vi "Actor Core.vi"(8 "error in":errorcluster, 11 "UI Main in":refnum<class "UI Main.lvclass">) -> (0 "error out":errorcluster, 3 "Actor out":refnum<class "Actor.lvclass">)   [LabVIEW 2020, in "UI Main.lvlib" / "UI Main.lvclass"]
doc: "(<B>Filename</B>: Actor Framework.lvlib:Actor.lvclass:Actor Core.vi)\n\nReceives messages to the actor, reacts to them, and initiates any error handling that may shut the actor down.\n\nDescendant classes may override this VI to append parallel tasks for the actor to complete while it handles messages. Overrides use the Call Parent Class Method node."
uses:
  UI Main.lvclass
  C:/Program Files (x86)/National Instruments/LabVIEW 2020/vi.lib/ActorFramework/Actor/Actor.lvclass
  <vilib>/ActorFramework/Actor/Actor.lvclass
  UI Status/UI Status/UI Status.lvclass
  UI Main Startup/UI Main Startup/UI Main Startup.lvclass
  <vilib>/ActorFramework/Actor/Actor.lvclass/Actor.ctl
  <vilib>/ActorFramework/Message Enqueuer/Message Enqueuer.lvclass/Message Enqueuer.ctl
  UI Main.lvclass/UI Main.ctl
  <vilib>/ActorFramework/Message Enqueuer/Init from Existing Queue.vi
  <vilib>/ActorFramework/Message Enqueuer/Enqueue.vi
  <vilib>/ActorFramework/Stop Msg/Stop Msg.lvclass
  C:/Program Files (x86)/National Instruments/LabVIEW 2020/vi.lib/ActorFramework/Message/Message.lvclass
  <vilib>/ActorFramework/Message Priority Queue/Priority Enqueue.vi
  <vilib>/ActorFramework/Message Enqueuer/Message Enqueuer.lvclass
  C:/git/Personal/Sandbox/ActorProject/UI Main/UI Main/UI Main.lvclass
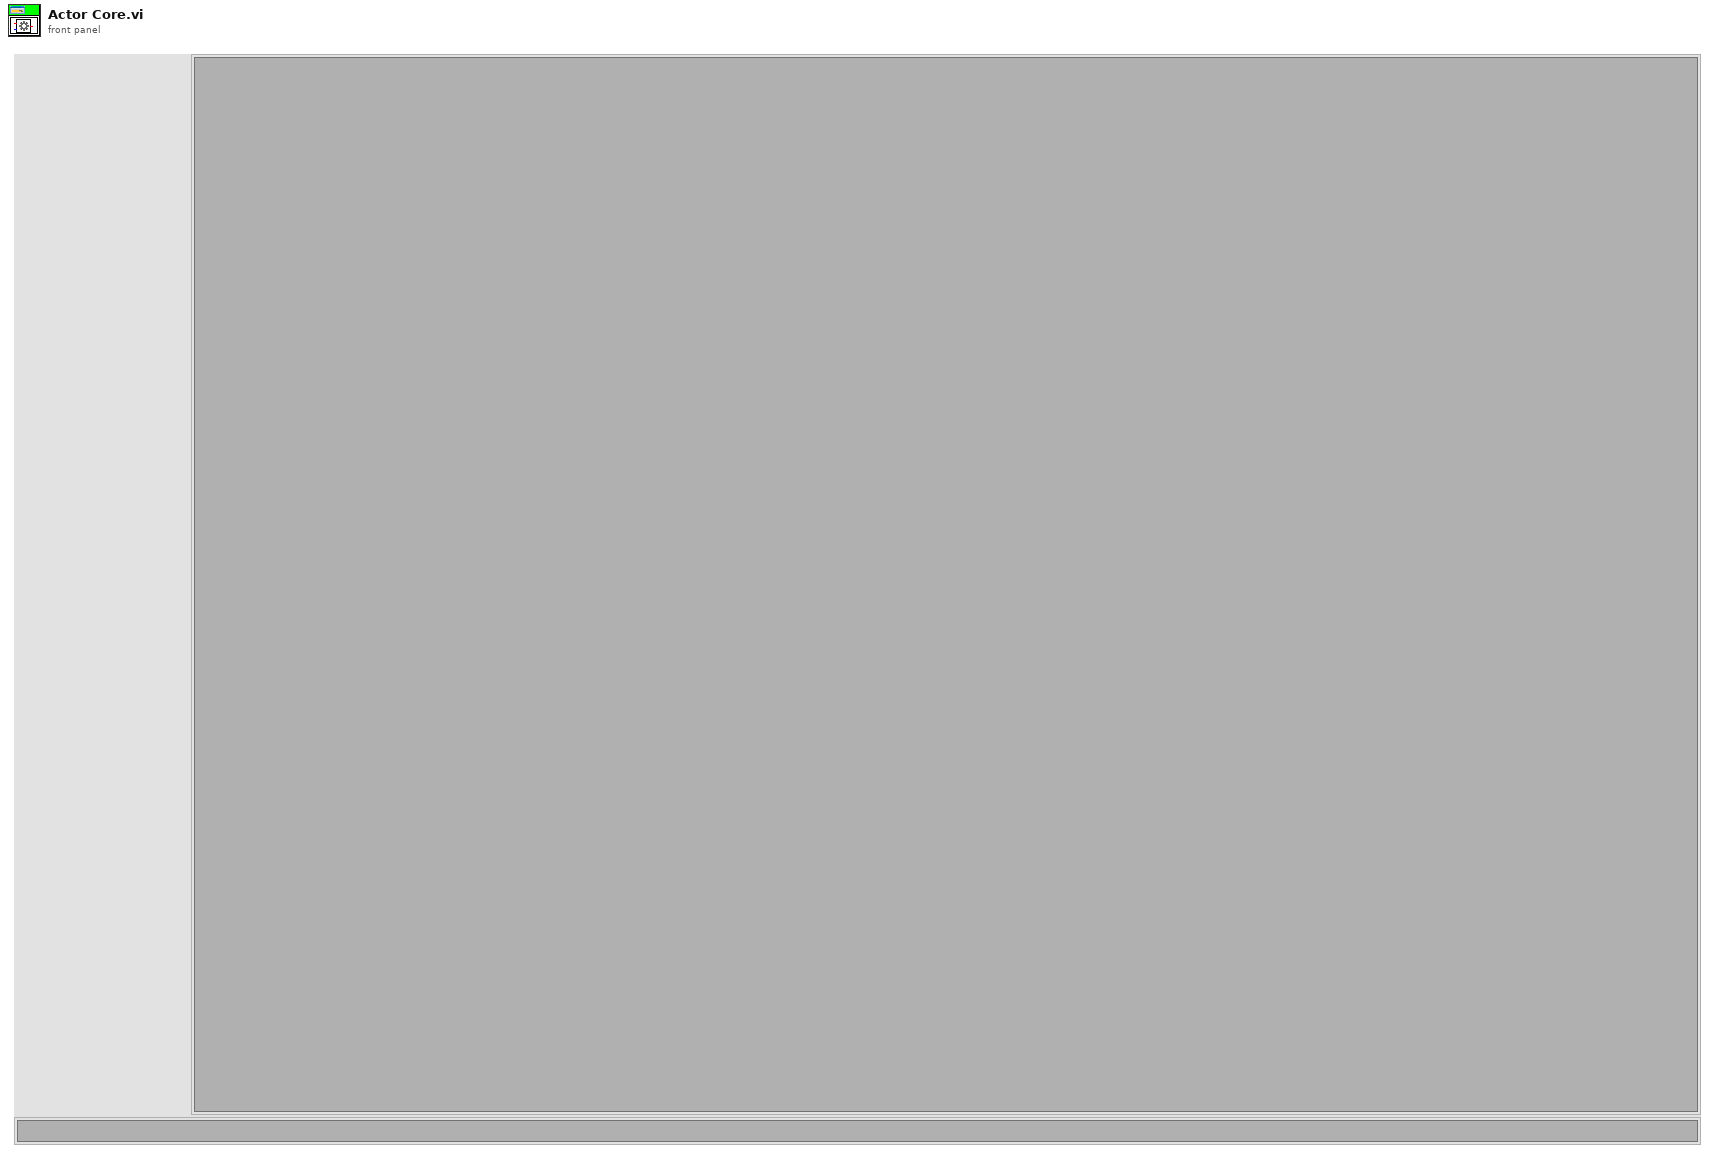
[diagram p1: front panel]
types:
  T1 = enum32{"Invalid", "Standard", "Closed", "Hidden", "Minimized", "Maximized"}
  T2 = cluster{"Stop":refnum<user-event>, "Sub Panel":refnum<user-event>}
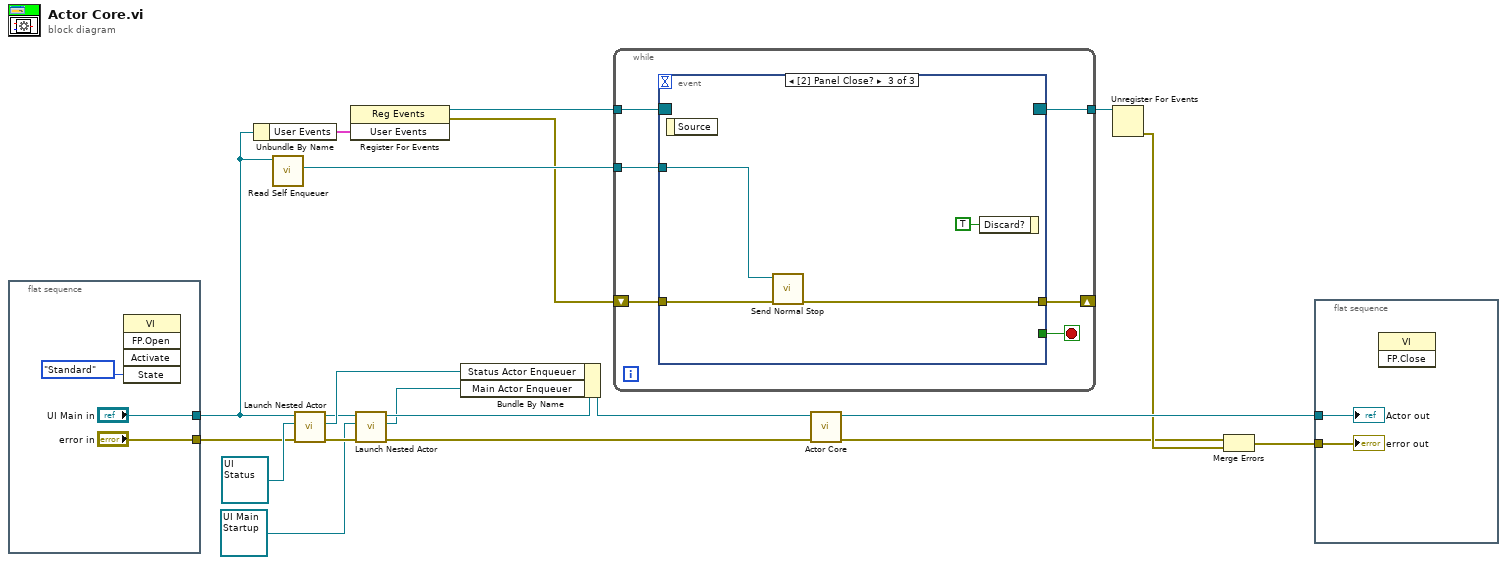
[diagram p0: block diagram]
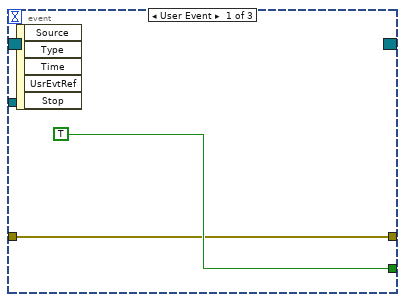
[diagram p2: hidden frame]
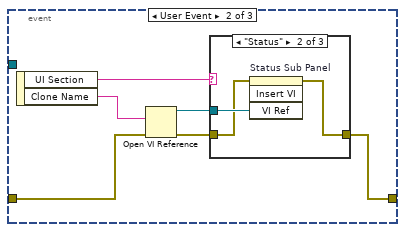
[diagram p3: hidden frame]
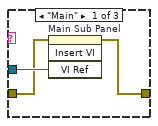
[diagram p4: hidden frame]
diagram:
  n1 = flat-sequence {
    tunnel: ["error in"] -> w16
    tunnel: ["UI Main in"] -> w9
    frame #0 {
      n2 = invoke class="VI" method="FP.Open"("State"=T1."Standard") -> ()  [unwired: 4 in, 5 out]
    }
  }
  n3 = Unbundle By Name(w9) -> ("User Events"=w15:T2)
  n4 = call <vilib>:"Read Self Enqueuer.vi"("Actor"=w9) -> ("Self Enqueuer"=w8:refnum<class "Message Enqueuer.lvclass">)  [unwired: 10 in]
  n5 = call <vilib>:"Launch Nested Actor.vi"("error in (no error)"=w16, "Nested Actor"=refnum<class "UI Status.lvclass"> refnum ("UI Status.lvlib:UI Status.lvclass"), "Caller Actor in"=w9) -> ("error out"=w4:errorcluster, "Nested Actor's Enqueuer"=w17:refnum<class "Message Enqueuer.lvclass">, "Caller Actor out"=w6:refnum<class "UI Main.lvclass">)  [unwired: 6 in]
  n6 = register-events(w15) -> (reference out=w14:refnum<event-registration>, error out=w7:errorcluster)  [unwired: 2 in]
  n7 = call <vilib>:"Launch Nested Actor.vi"("error in (no error)"=w4, "Nested Actor"=refnum<class "UI Main Startup.lvclass"> refnum ("UI Main Startup.lvlib:UI Main Startup.lvclass"), "Caller Actor in"=w6) -> ("error out"=w3:errorcluster, "Nested Actor's Enqueuer"=w1:refnum<class "Message Enqueuer.lvclass">, "Caller Actor out"=w5:refnum<class "UI Main.lvclass">)  [unwired: 6 in]
  n8 = Bundle By Name(cluster=w5, "Status Actor Enqueuer"=w17, "Main Actor Enqueuer"=w1) -> (w18:refnum<class "UI Main.lvclass">)
  n9 = while {
    tunnel: w14 -> [w29]
    tunnel: [w28] -> w13
    tunnel: w8 -> [w27]
    shift-right: [w24] -> _
    shift-left: w7 -> [w25]
    stop <- w26 stop-if-true
    n10 = event shown="[2] Panel Close?" {
      selector: w29 -> [_ _ _]
      dyn-events: [_ _ _] -> w28
      timeout: _ -> [_ _ _]
      tunnel: w27 -> [_ _ w45]
      tunnel: [TRUE _ _] -> w26
      tunnel: w25 -> [w30 w32 w46]
      tunnel: [w30 w33 w47] -> w24
      event User Event {
        n11 = event-data() -> ()  [unwired: 1 in, 5 out]
      }
      event User Event {
        n12 = event-data() -> ("UI Section"=w37:string, "Clone Name"=w36:string)  [unwired: 1 in]
        n13 = Open VI Reference(vi path=w36, error in (no error)=w32) -> (vi reference=w35:refnum<vi>, error out=w34:errorcluster)  [unwired: 4 in]
        n14 = case shown="\"Status\"" w37 {
          tunnel: w35 -> [w40 w43 _]
          tunnel: w34 -> [w39 w42 w44]
          tunnel: [w38 w41 w44] -> w33
          frame "Main" {
            n15 = invoke on="Main Sub Panel" class="SubPnl" method="Insert VI"(error in=w39, "VI Ref"=w40) -> (error out=w38:errorcluster)  [unwired: 2 in, 3 out]
          }
          frame "Status" {
            n16 = invoke on="Status Sub Panel" class="SubPnl" method="Insert VI"(error in=w42, "VI Ref"=w43) -> (error out=w41:errorcluster)  [unwired: 2 in, 3 out]
          }
          frame Default {
          }
        }
      }
      event Panel Close? {
        n17 = event-data() -> ()  [unwired: 1 in, 1 out]
        n18 = call <vilib>:"Send Normal Stop.vi"("error in (no error)"=w46, "Message Enqueuer"=w45) -> ("error out"=w47:errorcluster)  [unwired: 9 in]
        n19 = event-data("Discard?"=TRUE) -> ()  [unwired: 1 in, 1 out]
      }
    }
  }
  n20 = call-parent "Actor Core.vi"("error in"=w3, "Actor in"=w18) -> ("error out"=w11:errorcluster, "Actor out"=w20:refnum<class "Actor.lvclass">)  [unwired: 8 in]
  n21 = Unregister For Events(event registration refnum=w13) -> (error out=w12:errorcluster)  [unwired: 1 in]
  n22 = Merge Errors(w11, w12) -> (w10:errorcluster)
  n23 = flat-sequence {
    tunnel: w10 -> [w50]
    tunnel: w20 -> [w49]
    frame #0 {
      n24 = invoke class="VI" method="FP.Close"() -> ()  [unwired: 3 in, 3 out]
      "error out" <- w50
      "Actor out" <- w49
    }
  }
